vi "Run_Core.vi"(0 "For Loop in":refnum<class "While Loop.lvclass">, 11 "error in (no error)":errorcluster) -> (4 "For Loop out":refnum<class "While Loop.lvclass">, 6 "Return":variant, 15 "error out":errorcluster)   [LabVIEW 2016, in "While Loop.lvclass"]
uses:
  While Loop.lvclass
  D:/TOOLS/Funtion_Lists/source code/LSL components/functions/functionsbase/functionbase.lvclass
  functionsbase/functionbase.lvclass/functionbase.ctl
  functionsbase/properties/Read Smart Syntax Representation.vi
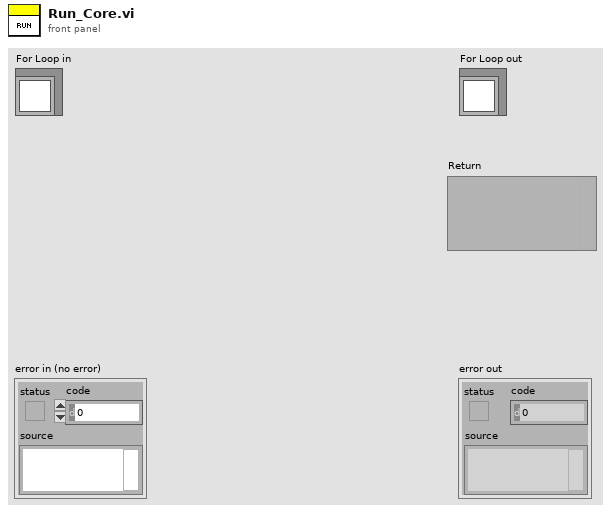
[diagram p1: front panel]
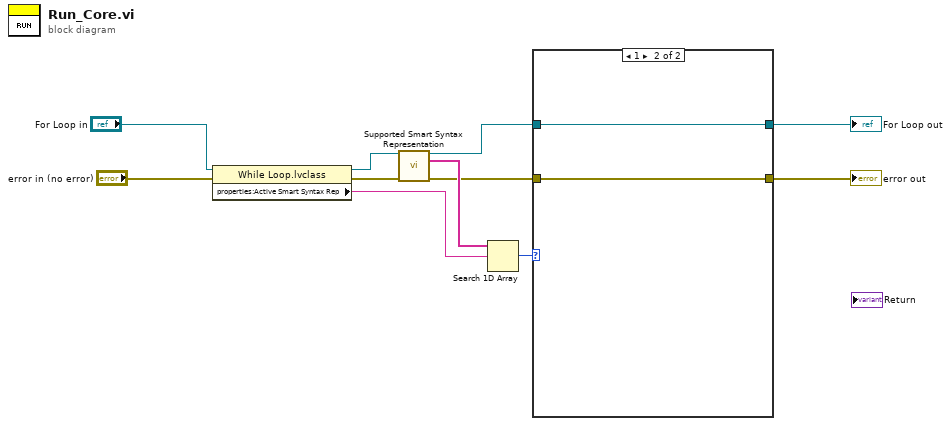
[diagram p0: block diagram]
diagram:
  n1 = property class="While Loop.lvclass"(reference="For Loop in", error in="error in (no error)") -> (reference out=w7:refnum<class "While Loop.lvclass">, error out=w10:errorcluster, "properties:Active Smart Syntax Rep"=w5:string)
  n2 = call-dynamic "Supported Smart Syntax Representation.vi"("For Loop in"=w7, "error in (no error)"=w10) -> ("For Loop out"=w4:refnum<class "While Loop.lvclass">, "Smart Syntax Representation List"=w9:string[], "error out"=w2:errorcluster)  [unwired: 11 in]
  n3 = Search 1D Array(1D array=w9, element=w5) -> (index of element=w8:i32)  [unwired: 1 in]
  n4 = case shown="1" w8 {
    tunnel: w4 -> [w13 w15]
    tunnel: [w13 w15] -> w3
    tunnel: w2 -> [w12 w14]
    tunnel: [w12 w14] -> w1
    frame 0, Default {
    }
    frame 1 {
    }
  }
  "error out" <- w1
  "For Loop out" <- w3
